vi "Actor Core.vi"(8 "error in":errorcluster, 11 "Nested in":refnum<class "User Interface.lvclass">) -> (0 "error out":errorcluster, 3 "Actor out":refnum<class "Actor.lvclass">)   [LabVIEW 2020, in "User Interface.lvlib" / "User Interface.lvclass"]
doc: "(<B>Filename</B>: Actor Framework.lvlib:Actor.lvclass:Actor Core.vi)\n\nReceives messages to the actor, reacts to them, and initiates any error handling that may shut the actor down.\n\nDescendant classes may override this VI to append parallel tasks for the actor to complete while it handles messages. Overrides use the Call Parent Method node."
uses:
  User Interface.lvclass
  C:/Program Files (x86)/National Instruments/LabVIEW 2020/vi.lib/ActorFramework/Actor/Actor.lvclass
  <vilib>/ActorFramework/Actor/Actor.lvclass
  Paquetes Disponibles/Paquetes Disponibles.lvclass
  Manejo Turnos/Manejo Turnos.lvclass
  Dinero/Dinero.lvclass
  <vilib>/ActorFramework/Actor/Actor.lvclass/Actor.ctl
  <vilib>/ActorFramework/Message Enqueuer/Message Enqueuer.lvclass/Message Enqueuer.ctl
  User Interface.lvclass/User Interface.ctl
  Dinero/Dinero.lvclass/Dinero.ctl
  Manejo Turnos/Manejo Turnos.lvclass/Manejo Turnos.ctl
  Paquetes Disponibles/Paquetes Disponibles.lvclass/Paquetes Disponibles.ctl
  <vilib>/ActorFramework/Message Enqueuer/Init from Existing Queue.vi
  <vilib>/ActorFramework/Message Enqueuer/Enqueue.vi
  <vilib>/ActorFramework/Stop Msg/Stop Msg.lvclass
  C:/Program Files (x86)/National Instruments/LabVIEW 2020/vi.lib/ActorFramework/Message/Message.lvclass
  User Interface Messages/Contabilidad Msg/Contabilidad Msg.lvclass
  <vilib>/ActorFramework/Message Priority Queue/Priority Enqueue.vi
  <vilib>/ActorFramework/Message Enqueuer/Message Enqueuer.lvclass
panel:
  in  "Contabilidad":bool
  in  "Stop":bool
  in  "Pausa":bool
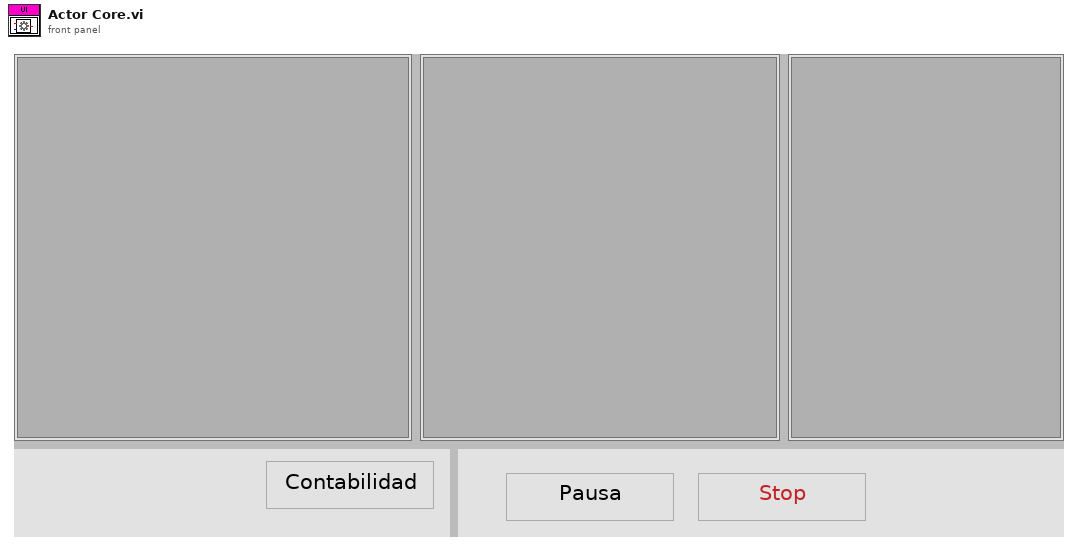
[diagram p1: front panel]
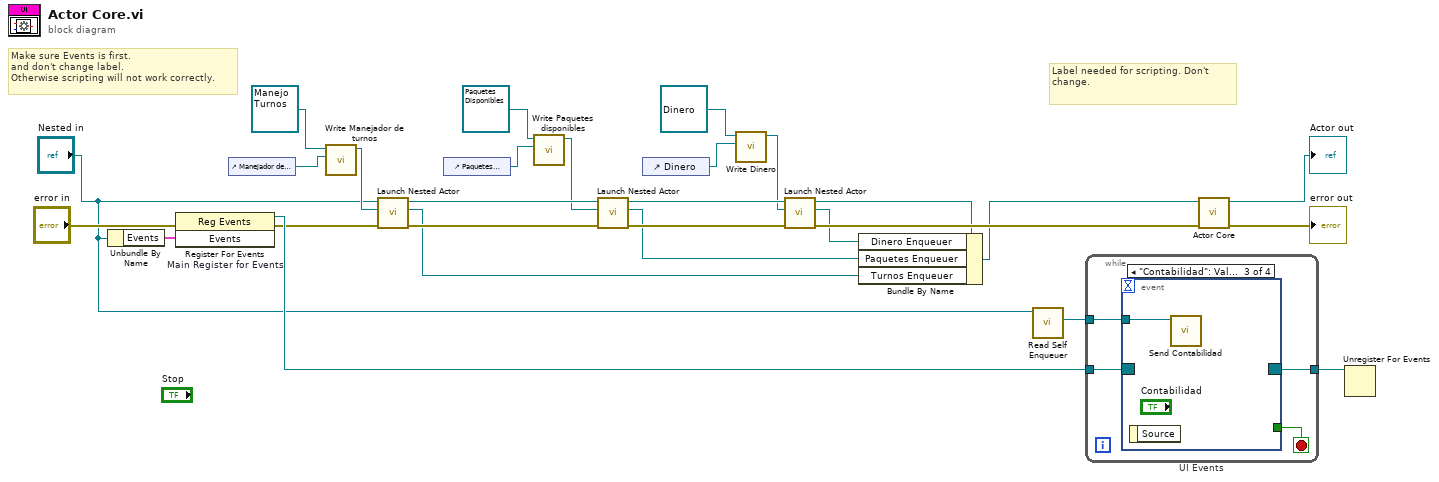
[diagram p0: block diagram]
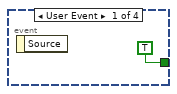
[diagram p2: hidden frame]
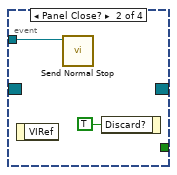
[diagram p3: hidden frame]
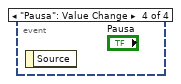
[diagram p4: hidden frame]
diagram:
  # "Label needed for scripting. Don't change."
  # "Make sure Events is first.\nand don't change label.\nOtherwise scripting will not work correctly."
  n1 = Unbundle By Name("Nested in") -> ("Events"=w25:cluster{"Stop":refnum<user-event>})
  n2 = register-events "Main Register for Events"(error in="error in", w25) -> (reference out=w26:refnum<event-registration>, error out=w21:errorcluster)  [unwired: 1 in]
  n3 = control-ref of="Manejador de turnos"() -> (w3:refnum<vi>)
  n4 = call "Write Manejador de turnos.vi"("Manejador de turnos"=w3, "Manejo Turnos in"=refnum<class "Manejo Turnos.lvclass"> refnum ("Manejo Turnos.lvlib:Manejo Turnos.lvclass")) -> ("Manejo Turnos out"=w2:refnum<class "Manejo Turnos.lvclass">)  [unwired: 8 in, 1 out]
  n5 = call <vilib>:"Launch Nested Actor.vi"("error in (no error)"=w21, "Nested Actor"=w2, "Caller Actor in"="Nested in") -> ("error out"=w16:errorcluster, "Nested Actor's Enqueuer"=w13:refnum<class "Message Enqueuer.lvclass">, "Caller Actor out"=w11:refnum<class "User Interface.lvclass">)  [unwired: 6 in]
  n6 = control-ref of="Paquetes disponibles"() -> (w8:refnum<vi>)
  n7 = call "Write Paquetes disponibles.vi"("Paquetes disponibles"=w8, "Paquetes Disponibles in"=refnum<class "Paquetes Disponibles.lvclass"> refnum ("Paquetes Disponibles.lvlib:Paquetes Disponibles.lvclass")) -> ("Paquetes Disponibles out"=w10:refnum<class "Paquetes Disponibles.lvclass">)  [unwired: 8 in, 1 out]
  n8 = call <vilib>:"Launch Nested Actor.vi"("error in (no error)"=w16, "Nested Actor"=w10, "Caller Actor in"=w11) -> ("error out"=w19:errorcluster, "Nested Actor's Enqueuer"=w14:refnum<class "Message Enqueuer.lvclass">, "Caller Actor out"=w18:refnum<class "User Interface.lvclass">)  [unwired: 6 in]
  n9 = control-ref of="Dinero"() -> (w5:refnum<vi>)
  n10 = call "Write Dinero.vi"("Dinero"=w5, "Dinero in"=refnum<class "Dinero.lvclass"> refnum ("Dinero.lvlib:Dinero.lvclass")) -> ("Dinero out"=w7:refnum<class "Dinero.lvclass">)  [unwired: 8 in, 1 out]
  n11 = call <vilib>:"Launch Nested Actor.vi"("error in (no error)"=w19, "Nested Actor"=w7, "Caller Actor in"=w18) -> ("error out"=w20:errorcluster, "Nested Actor's Enqueuer"=w15:refnum<class "Message Enqueuer.lvclass">, "Caller Actor out"=w17:refnum<class "User Interface.lvclass">)  [unwired: 6 in]
  n12 = Bundle By Name(cluster=w17, "Dinero Enqueuer"=w15, "Paquetes Enqueuer"=w14, "Turnos Enqueuer"=w13) -> (w12:refnum<class "User Interface.lvclass">)
  n13 = call <vilib>:"Read Self Enqueuer.vi"("Actor"="Nested in") -> ("Self Enqueuer"=w23:refnum<class "Message Enqueuer.lvclass">)  [unwired: 10 in]
  n14 = while {
    tunnel: w26 -> [w32]
    tunnel: [w30] -> w24
    tunnel: w23 -> [w29]
    stop <- w31 stop-if-true
    n15 = event "UI Events" shown="[2] \"Contabilidad\": Value Change" {
      selector: w32 -> [_ _ _ _]
      dyn-events: [_ _ _ _] -> w30
      timeout: _ -> [_ _ _ _]
      tunnel: [TRUE _ _ _] -> w31
      tunnel: w29 -> [_ w34 w36 _]
      event User Event {
        n16 = event-data() -> ()  [unwired: 1 in, 1 out]
      }
      event Panel Close? {
        n17 = event-data() -> ()  [unwired: 1 in, 1 out]
        n18 = call <vilib>:"Send Normal Stop.vi"("Message Enqueuer"=w34) -> ()  [unwired: 10 in, 1 out]
        n19 = event-data("Discard?"=TRUE) -> ()  [unwired: 1 in, 1 out]
      }
      event "Contabilidad": Value Change {
        n20 = event-data() -> ()  [unwired: 1 in, 1 out]
        n21 = call "Send Contabilidad.vi"("Message Enqueuer"=w36) -> ()  [unwired: 9 in, 2 out]
      }
      event "Pausa": Value Change {
        n22 = event-data() -> ()  [unwired: 1 in, 1 out]
      }
    }
  }
  n23 = call-parent "Actor Core.vi"("error in"=w20, "Actor in"=w12) -> ("error out"=→"error out":errorcluster, "Actor out"=→"Actor out":refnum<class "Actor.lvclass">)  [unwired: 8 in]
  n24 = Unregister For Events(event registration refnum=w24) -> ()  [unwired: 1 in, 1 out]
